vi "_Parse SEM Segment Limit Check Result.vi"(8 "error in (no error)":errorcluster, 10 "Input String":string, 11 "VISA resource name":refnum<visa-resource-name>) -> (0 "error out":errorcluster, 1 "SEM Limit Check Results":cluster{"OBW":i32, "TX Power":i32}, 2 "Reliability Results":T1, 3 "VISA resource name out":refnum<visa-resource-name>, 5 "Out Of Tolerance":dbl format="%^.3e", 7 "Statistic Expired":i32)   [LabVIEW 2020, in "Rohde&Schwarz CMXP NR FR2 Measurement.lvlib"]
uses:
  <instrlib>/Rohde&Schwarz CMXP NR FR2 Measurement/Rohde&Schwarz CMXP NR FR2 Measurement.lvlib
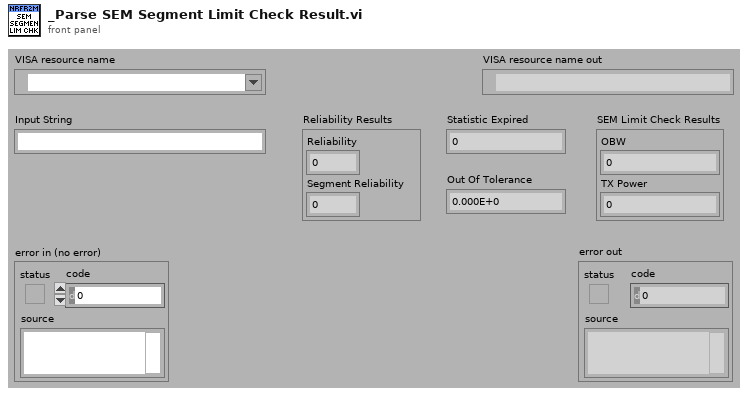
[diagram p1: front panel]
types:
  T1 = cluster{"Reliability":i32, "Segment Reliability":i32}
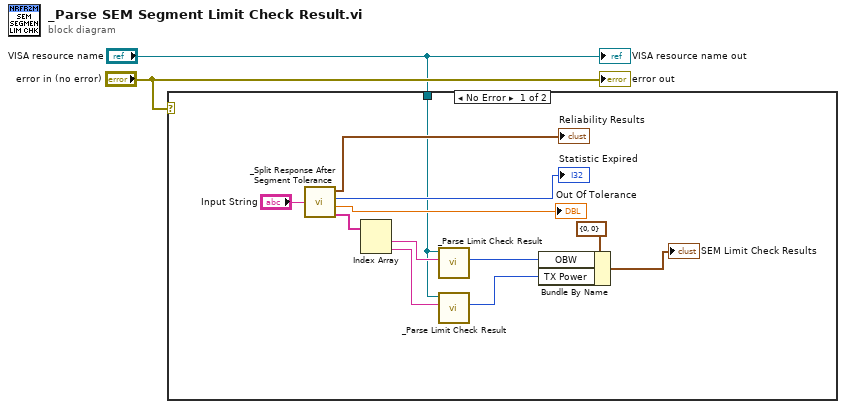
[diagram p0: block diagram]
diagram:
  n1 = case shown="No Error" "error in (no error)" {
    tunnel: "VISA resource name" -> [w3 _]
    frame No Error {
      n2 = call <instrlib>:"_Split Response After Segment Tolerance.vi"("Input String"="Input String") -> ("Reliability Results"=→"Reliability Results":T1, "Statistic Expired"=→"Statistic Expired":i32, "Out Of Tolerance"=→"Out Of Tolerance":dbl, "Response out"=w12:string[])
      n3 = Index Array(array=w12) -> (element #1=w11:string, element #2=w10:string)  [unwired: 2 in]
      n4 = call <instrlib>:"_Parse Limit Check Result.vi"("String Value In"=w11, "VISA resource name"=w3) -> ("Limit Check Value"=w14:i32)  [unwired: 7 in, 2 out]
      n5 = call <instrlib>:"_Parse Limit Check Result.vi"("String Value In"=w10, "VISA resource name"=w3) -> ("Limit Check Value"=w9:i32)  [unwired: 7 in, 2 out]
      n6 = Bundle By Name(cluster=cluster{"OBW":i32, "TX Power":i32} {"OBW"=0, "TX Power"=0} ("SEM Results"), "OBW"=w14, "TX Power"=w9) -> (→"SEM Limit Check Results":cluster{"OBW":i32, "TX Power":i32})
    }
    frame Error {
    }
  }
  "error out" <- "error in (no error)"
  "VISA resource name out" <- "VISA resource name"
